vi "循环时状态显示 - 3.vi"(8 "Str引用句柄":refnum<vi>, 9 "cmd:":string, 10 "新信息输入":string) -> ()   [LabVIEW 2017]
uses:
  Global System.vi
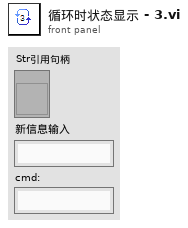
[diagram p1: front panel]
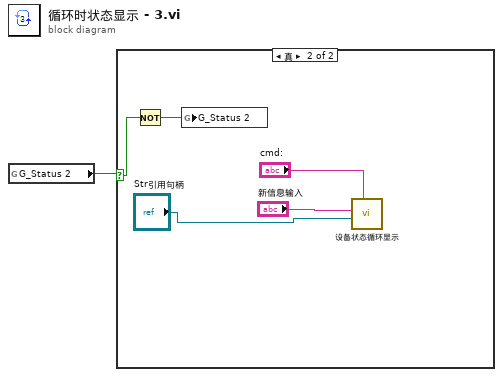
[diagram p0: block diagram]
diagram:
  n1 = global read "Global System.vi" "G_Status 2"() -> (w1:bool)
  n2 = case shown="真" w1 {
    selector: w1 -> [_ w6]
    frame False {
    }
    frame True {
      n3 = Not(x=w6) -> (.not. x?=w2:bool)
      n4 = global write "Global System.vi" "G_Status 2"(w2) -> ()
      n5 = call "设备状态循环显示.vi"("cmd:"="cmd:", "Str引用句柄"="Str引用句柄", "新信息输入"="新信息输入") -> ()  [unwired: 9 in]
    }
  }
